vi "Camera_Sim_Create.vi"(0 "reference in":refnum<class "Camera_Sim.lvclass">, 5 "Simulated Image Directory":path, 11 "error in (no error)":errorcluster) -> (4 "reference out":refnum<class "Camera_Sim.lvclass">, 15 "error out":errorcluster)   [LabVIEW 2017, in "Camera_Sim.lvclass"]
uses:
  Camera_Sim.lvclass
  C:/VIT/simpleImageProcessingExample/lv_src/Camera/Camera_class/Camera.lvclass
  <vilib>/vision/Image Controls.llb/IMAQ Image.ctl
  Camera_class/Camera.lvclass
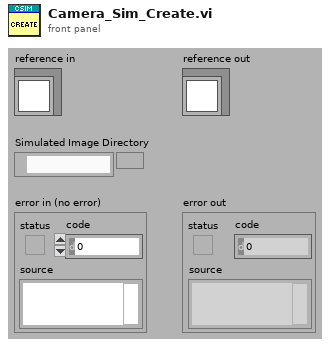
[diagram p1: front panel]
types:
  T1 = typedef "IMAQ Image.ctl" = refnum<image>
  T2 = typedef "Camera_Sim.lvclass/ObjectAttributes.ctl" = cluster{"Connected":bool, "Image Out":T1, "Frame Number":u32, "Image Directory":path, "Images in Directory":path[]}
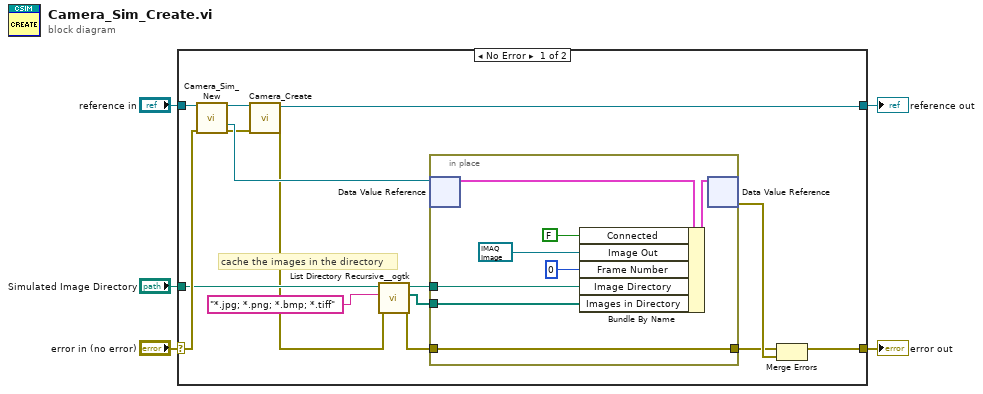
[diagram p0: block diagram]
diagram:
  n1 = case shown="No Error" "error in (no error)" {
    selector: "error in (no error)" -> [w18 w30]
    tunnel: [w16 w30] -> w4
    tunnel: "reference in" -> [w19 w29]
    tunnel: [w13 w29] -> w2
    tunnel: "Simulated Image Directory" -> [w11 _]
    frame No Error {
      # "cache the images in the directory"
      n2 = call "Camera_Sim_New.vi"("reference in"=w19, "error in (no error)"=w18) -> ("reference out"=w14:refnum<class "Camera_Sim.lvclass">, "DVRRefOut"=w20:refnum<data-value>, "error out"=w12:errorcluster)  [unwired: 10 in, 1 out]
      n3 = call "Camera_Create.vi"("error in (no error)"=w12, "reference in"=w14) -> ("error out"=w9:errorcluster, "reference out"=w13:refnum<class "Camera_Sim.lvclass">)  [unwired: 8 in]
      n4 = call <userlib>:"List Directory Recursive__ogtk.vi"("error in (no error)"=w9, "pattern"="*.jpg; *.png; *.bmp; *.tiff", "Path"=w11) -> ("error out"=w8:errorcluster, "file paths"=w7:path[], "dup Path"=w10:path)  [unwired: 5 in, 1 out]
      n5 = in-place {
        in-place-border: w8 -> [w26]
        in-place-border: [w26] -> w15
        in-place-border: w10 -> [w22]
        in-place-border: w7 -> [w21]
        n6 = in-place-dvr #1(w20) -> (w27:T2)  [unwired: 1 out]
        n7 = Bundle By Name(cluster=w27, "Connected"=FALSE, "Image Out"=T1 refnum, "Frame Number"=u32 0, "Image Directory"=w22, "Images in Directory"=w21) -> (w28:T2)
        n8 = in-place-dvr #1(w28) -> (w17:errorcluster)  [unwired: 1 out]
      }
      n9 = Merge Errors(w15, w17) -> (w16:errorcluster)
    }
    frame Error {
    }
  }
  "error out" <- w4
  "reference out" <- w2
